vi "GetType.vi"(8 "error in (no error)":errorcluster, 11 "Get Aperture Time Info [DT] Msg":refnum<class "Get Aperture Time Info [DT] Msg.lvclass">) -> (0 "error out":errorcluster, 2 "Data Sample":variant, 3 "Get Aperture Time Info [DT] Msg":refnum<class "Get Aperture Time Info [DT] Msg.lvclass">)   [LabVIEW 2016, in "CS++DMM.lvlib" / "Get Aperture Time Info [DT] Msg.lvclass"]
uses:
  Get Aperture Time Info [DT] Msg.lvclass
  Get Aperture Time Info [DT] Msg.lvclass/Get Aperture Time Info [DT] Msg.ctl
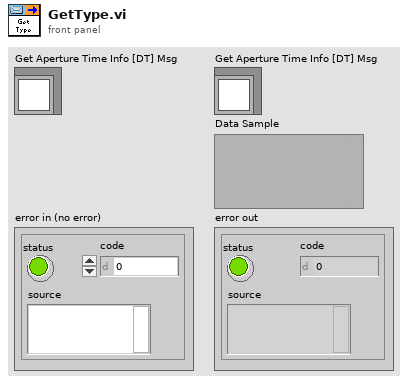
[diagram p1: front panel]
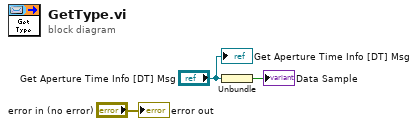
[diagram p0: block diagram]
diagram:
  n1 = Unbundle("Get Aperture Time Info [DT] Msg") -> (→"Data Sample":bool)
  "error out" <- "error in (no error)"
  "Get Aperture Time Info [DT] Msg" <- "Get Aperture Time Info [DT] Msg"
